vi "Untitled 3.vi"(11 "Message Cluster":T1) -> (3 "Message Cluster 2":T1)   [LabVIEW 2017]
uses:
  Message Queue/Message Cluster.ctl
  Message Queue/Message Queue.lvlib
panel:
  in  "s":bool
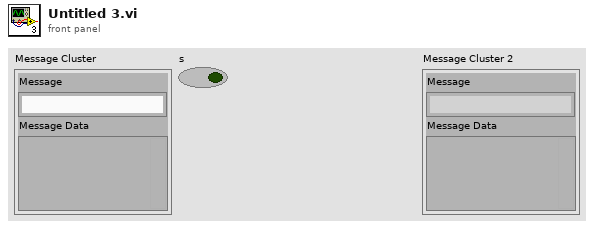
[diagram p1: front panel]
types:
  T1 = typedef "Message Queue.lvlib/Message Cluster.ctl" = cluster{"Message":string, "Message Data":variant}
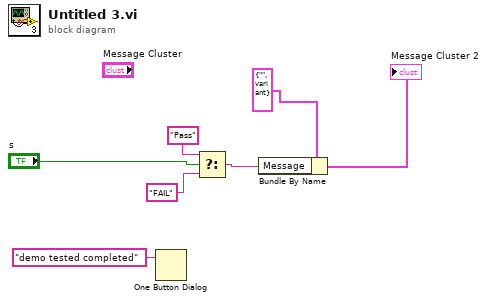
[diagram p0: block diagram]
diagram:
  n1 = One Button Dialog(message="demo tested completed") -> ()  [unwired: 1 in, 1 out]
  n2 = Select(t="Pass" ("Message"), s="s", f="FAIL") -> (s? t:f=w2:string)
  n3 = Bundle By Name(cluster=T1 {"Message"="", "Message Data"=variant} ("Message Cluster"), "Message"=w2) -> (→"Message Cluster 2":T1)
